vi "Init FPGA code.vi"(8 "error in (no error)":errorcluster, 11 "Device Ref in":T1 format="%.0x") -> (0 "Error out":errorcluster, 1 "DMA FIFO ref":refnum<k20>, 2 "Bitfile ref":refnum<k20>, 3 "Device Ref out":T1 format="%.0x")   [LabVIEW 2014, in "SLSC configuration Engine.lvlib"]
uses:
  SLSC configuration Engine.lvlib
  <vilib>/NI Veristand/Custom Device API/Custom Device Item Ref.ctl
  <vilib>/NI Veristand/Custom Device API/Custom Device API.lvlib
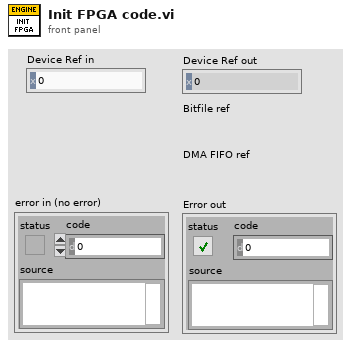
[diagram p1: front panel]
types:
  T1 = typedef "Custom Device API.lvlib/Custom Device Item Ref.ctl" = u64
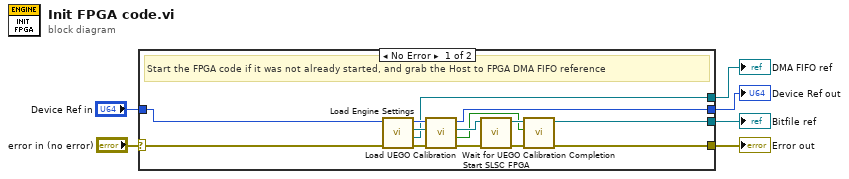
[diagram p0: block diagram]
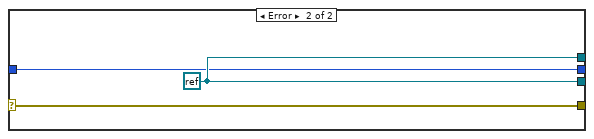
[diagram p2: hidden frame]
diagram:
  n1 = case shown="No Error" "error in (no error)" {
    selector: "error in (no error)" -> [w19 w22]
    tunnel: "Device Ref in" -> [w20 w21]
    tunnel: [w8 w23] -> w6
    tunnel: [w15 w23] -> w2
    tunnel: [w9 w22] -> w5
    tunnel: [w7 w21] -> w1
    frame No Error {
      # "Start the FPGA code if it was not already started, and grab the Host to FPGA DMA FIFO reference"
      n2 = call "Load Engine Settings.vi"("error in (no error)"=w19, "Device Ref in"=w20) -> ("error out"=w18:errorcluster, "FIFO Ref out"=w15:refnum<k20>, "FPGA Ref out"=w16:refnum<k20>, "Device Ref out"=w17:T1)  [unwired: 6 in]
      n3 = call "Load UEGO Calibration.vi"("error in (no error)"=w18, "FPGA Ref in"=w16, "Device Ref in"=w17) -> ("error out"=w13:errorcluster, "UEGO Present?"=w10:bool, "FPGA Ref out"=w14:refnum<k20>, "Device Ref out"=w7:T1)  [unwired: 5 in]
      n4 = call "Start SLSC FPGA.vi"("error in (no error)"=w13, "FPGA Ref in"=w14) -> ("error out"=w12:errorcluster, "FPGA Ref out"=w11:refnum<k20>)  [unwired: 8 in]
      n5 = call "Wait for UEGO Calibration Completion.vi"("error in"=w12, "UEGO Present?"=w10, "FPGA Ref in"=w11) -> ("error out"=w9:errorcluster, "FPGA Ref out"=w8:refnum<k20>)  [unwired: 7 in]
    }
    frame Error {
      w23 = refnum<k0> refnum
    }
  }
  "Bitfile ref" <- w6
  "Error out" <- w5
  "Device Ref out" <- w1
  "DMA FIFO ref" <- w2
